vi "solar_voy_def Import (Required).vi"(5 "Endian (BIG)":enum8{"BIG", "LITTLE"}(ring), 6 "Suppress Errors? (T)":bool=TRUE, 8 "error in (no error)":errorcluster, 11 "Target Name":string) -> (0 "error out":errorcluster, 3 "PACKETS (No HDR)":T1[](array[typedef]) {"last_time" format="%<%H:%M:%S%3u %m/%d/%y>T"})   [LabVIEW 2018]
doc: "This imports the required packets for the LINC interface. Required packets include: \nCOSMOS_ERROR_IGNORE\nCOSMOS_ERROR_HANDLE\nCOSMOS_HANDSHAKE_EN\nCOSMOS_HANDSHAKE_DS\nHANDSHAKE\nERROR"
uses:
  solar_voy_def_ctl ITEM TYPE.ctl
  type/solar_type Item Type.ctl
  solar_voy_def_ctl ITEM.ctl
  solar_voy_def_ctl PACKET_ID.ctl
  solar_voy_def_ctl PACKET.ctl
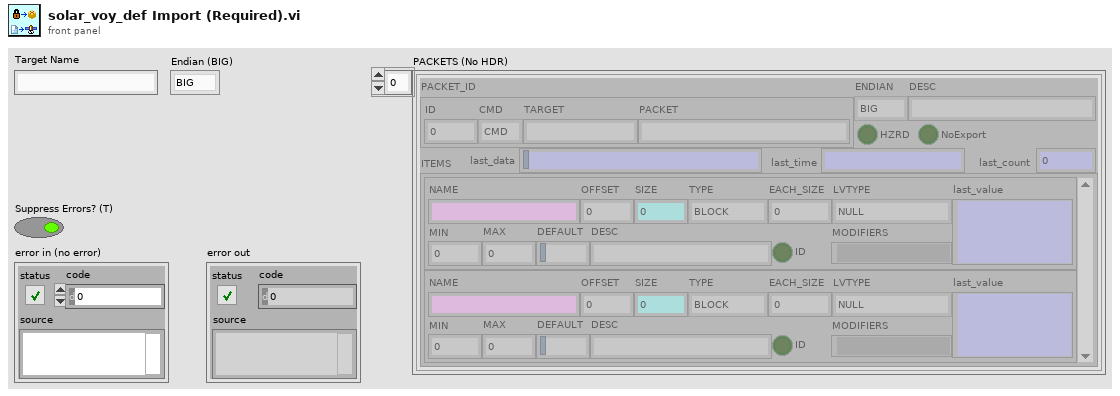
[diagram p1: front panel]
types:
  T1 = typedef "solar_voy_def_ctl PACKET.ctl" = cluster{"PACKET_ID":T2, "ENDIAN":enum8{"BIG", "LITTLE"}, "DESC":string, "HZRD":bool, "ITEMS":T3[], "NoExport":bool, "last_time":timestamp, "last_count":u32, "last_data":string}
  T2 = typedef "solar_voy_def_ctl PACKET_ID.ctl" = cluster{"ID":u16, "CMD":enum8{"CMD", "TLM"}, "TARGET":string, "PACKET":string}
  T3 = typedef "solar_voy_def_ctl ITEM.ctl" = cluster{"NAME":string, "OFFSET":i32, "SIZE":i32, "TYPE":T4, "EACH_SIZE":i32, "LVTYPE":T5, "MIN":dbl, "MAX":dbl, "DEFAULT":string, "DESC":string, "ID":bool, "MODIFIERS":variant, "last_value":variant}
  T4 = typedef "solar_voy_def_ctl ITEM TYPE.ctl" = enum8{"BLOCK", "INT", "UINT", "FLOAT", "STRING"}
  T5 = typedef "solar_type Item Type.ctl" = enum16{"NULL", "UNKNOWN", "CLUSTER", "I8", "I16", "I32", "I64", "U8", "U16", "U32", "U64", "U8_ENUM", "U16_ENUM", "U32_ENUM", "SGL", "DBL", "BOOLEAN", "STRING", "PATH", "VISA", "TAG", "TIME", "I8_1D", "I16_1D", "I32_1D", "I64_1D", "U8_1D", "U16_1D", "U32_1D", "U64_1D", "U8_ENUM_1D", "U16_ENUM_1D", "U32_ENUM_1D", "SGL_1D", "DBL_1D", "BOOLEAN_1D", "STRING_1D", "PATH_1D", "VISA_1D", "TAG_1D", "TIME_1D", "I8_2D", "I16_2D", "I32_2D", "I64_2D", "U8_2D", "U16_2D", "U32_2D", "U64_2D", "U8_ENUM_2D", "U16_ENUM_2D", "U32_ENUM_2D", "SGL_2D", "DBL_2D", "BOOLEAN_2D", "STRING_2D", "PATH_2D", "VISA_2D", "TAG_2D", "TIME_2D"}
  T6 = cluster{"ORIGIN":enum8{"RMT", "LCL"}, "STATUS,s=OK|ERROR":bool, "CODE":i32, "TIME_SECONDS":u32, "TIME_MICROSECONDS":u32, "DATA,t=BLOCK":string}
  T7 = cluster{"STATUS,s=OK|ERROR":bool, "CODE":i32, "SOURCE":string}
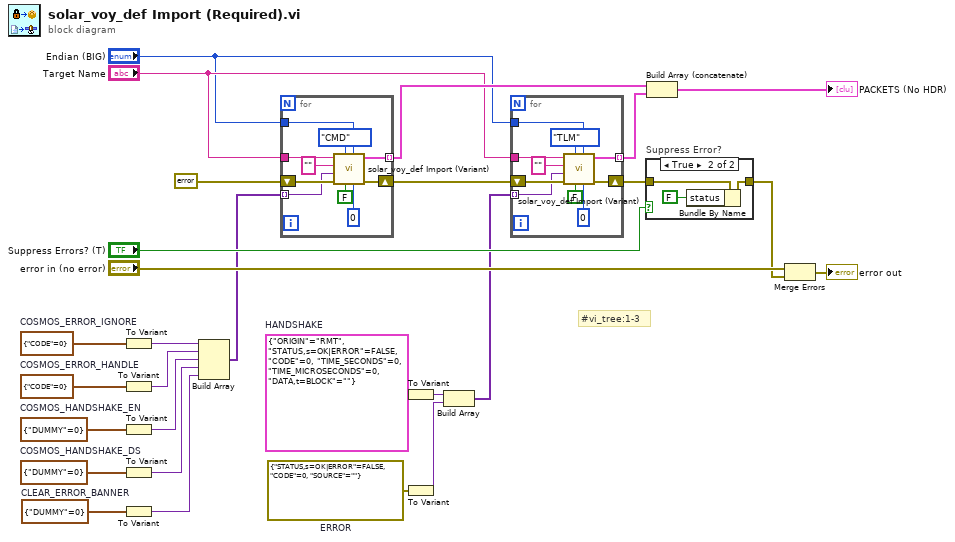
[diagram p0: block diagram]
diagram:
  w2 = cluster{"DUMMY":u8} {"DUMMY"=0}  # CLEAR_ERROR_BANNER
  w13 = T6 {"ORIGIN"=enum."RMT", "STATUS,s=OK|ERROR"=FALSE, "CODE"=0, "TIME_SECONDS"=0, "TIME_MICROSECONDS"=0, "DATA,t=BLOCK"=""}  # HANDSHAKE
  w16 = T7 {"STATUS,s=OK|ERROR"=FALSE, "CODE"=0, "SOURCE"=""}  # ERROR
  w20 = cluster{"DUMMY":u8} {"DUMMY"=0}  # COSMOS_HANDSHAKE_DS
  w21 = cluster{"DUMMY":u8} {"DUMMY"=0}  # COSMOS_HANDSHAKE_EN
  w22 = cluster{"CODE":i32} {"CODE"=0}  # COSMOS_ERROR_HANDLE
  w24 = cluster{"CODE":i32} {"CODE"=0}  # COSMOS_ERROR_IGNORE
  # "#vi_tree:1-3"
  n1 = To Variant(anything=w24) -> (Variant=w23:variant)
  n2 = To Variant(anything=w22) -> (Variant=w19:variant)
  n3 = To Variant(anything=w21) -> (Variant=w18:variant)
  n4 = To Variant(anything=w20) -> (Variant=w17:variant)
  n5 = To Variant(anything=w2) -> (Variant=w1:variant)
  n6 = Build Array(w23, w19, w18, w17, w1) -> (w3:variant[])
  n7 = for {
    tunnel: "Target Name" -> [w31]
    tunnel: w3 -> [w34] mode=indexing
    shift-right: [w37] -> w9
    shift-left: errorcluster {"status"=FALSE, "code"=0, "source"=""} ("error out") -> [w38]
    tunnel: [w35] -> w11 mode=indexing
    tunnel: "Endian (BIG)" -> [w30]
    n8 = call "solar_voy_def Import (Variant).vi"("Default ID"=u16 0, "Endian (BIG)"=w30, "Suppress Errors? (T)"=FALSE, "CMD"=enum8{"CMD", "TLM"}."CMD" ("TYPE"), "error in (no error)"=w38, "Variant"=w34, "PACKET (\"\"=Use Variant)"="" ("PACKET (\"\"=Use Variant)"), "TARGET"=w31) -> ("error out"=w37:errorcluster, "PACKET"=w35:T1)  [unwired: 2 in]
  }
  n9 = To Variant(anything=w13) -> (Variant=w15:variant)
  n10 = To Variant(anything=w16) -> (Variant=w14:variant)
  n11 = Build Array(w15, w14) -> (w8:variant[])
  n12 = for {
    tunnel: "Target Name" -> [w41]
    tunnel: w8 -> [w44] mode=indexing
    shift-right: [w47] -> w4
    shift-left: w9 -> [w48]
    tunnel: [w45] -> w5 mode=indexing
    tunnel: "Endian (BIG)" -> [w40]
    n13 = call "solar_voy_def Import (Variant).vi"("Default ID"=u16 0, "Endian (BIG)"=w40, "Suppress Errors? (T)"=FALSE, "CMD"=enum8{"CMD", "TLM"}."TLM" ("TYPE"), "error in (no error)"=w48, "Variant"=w44, "PACKET (\"\"=Use Variant)"="" ("PACKET (\"\"=Use Variant)"), "TARGET"=w41) -> ("error out"=w47:errorcluster, "PACKET"=w45:T1)  [unwired: 2 in]
  }
  n14 = case "Suppress Error?" shown="True" "Suppress Errors? (T)" {
    tunnel: w4 -> [w49 w52]
    tunnel: [w49 w51] -> w26
    frame False {
    }
    frame True {
      n15 = Bundle By Name(cluster=w52, "status"=FALSE) -> (w51:errorcluster)
    }
  }
  n16 = Build Array (concatenate)(w11, w5) -> (→"PACKETS (No HDR)":T1[])
  n17 = Merge Errors("error in (no error)", w26) -> (→"error out":errorcluster)
